vi "read_spectrometer.vi"() -> (0 "spectrometer_data":dbl[][](array[numeric]))   [LabVIEW 2018]
panel:
  out "falling":dbl
  out "FPWM":dbl
  out "rasing":dbl
  out "center wavelength":dbl
  in  "停止":bool
  out "XY Graph":cluster{"Y":dbl[], "Y":dbl[]}[](graph) caption="XY图"
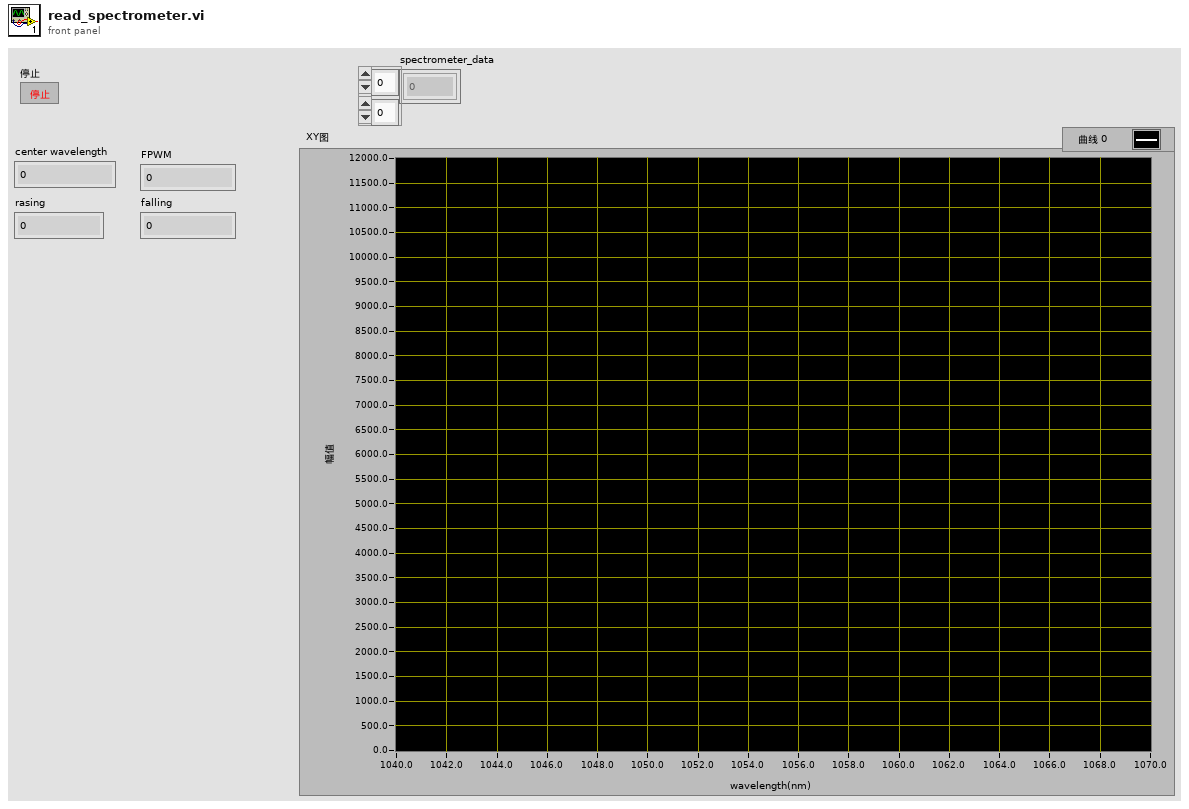
[diagram p1: front panel]
types:
  T1 = enum16{"Read", "Write", "ReadWrite", "BufferedRead", "BufferedReadWrite"}
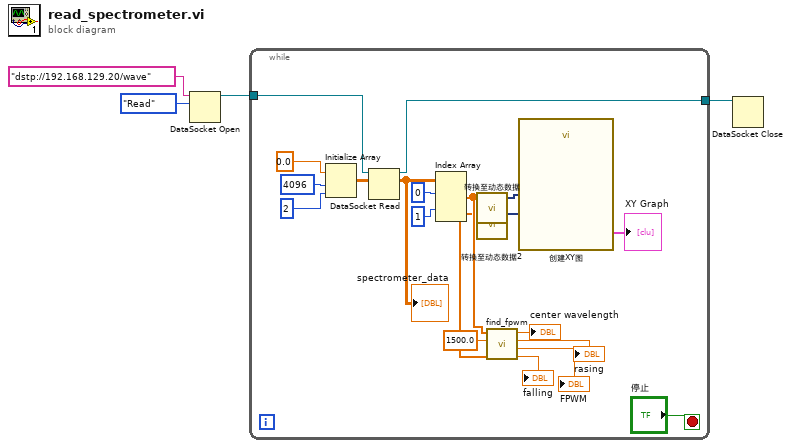
[diagram p0: block diagram]
diagram:
  n1 = DataSocket Open(10:T1."Read" ("模式"), 11:"dstp://192.168.129.20/wave" ("URL")) -> (3:w2:refnum<k13>)  [unwired: 2 in, 1 out]
  n2 = while {
    tunnel: w2 -> [w14]
    tunnel: [w12] -> w1
    stop <- "停止" stop-if-true
    n3 = Initialize Array(0.0 ("元素"), 4096 ("维数大小"), 2 ("维数大小")) -> (w21:dbl[][])
    n4 = DataSocket Read(10:w21, 11:w14) -> (2:w20:dbl[][], 3:w12:refnum<k13>)  [unwired: 3 in, 5 out]
    "spectrometer_data" <- w20
    n5 = Index Array(array=w20, index (row) #1=0 ("索引 (行)"), index (row) #2=1 ("索引 (行)")) -> (element #1=w11:dbl[], element #2=w10:dbl[])  [unwired: 2 in]
    n6 = call "转换至动态数据"("Array"=w11) -> ("Dynamic Data Type"=w16:dynamicdata)  [unwired: 3 in]
    n7 = call "转换至动态数据2"("Array"=w10) -> ("Dynamic Data Type"=w15:dynamicdata)  [unwired: 3 in]
    n8 = call "find_fpwm.vi"("Y"=w10, "baseline"=1500.0, "X"=w11) -> ("falling"=→"falling":dbl, "FPWM"=→"FPWM":dbl, "rasing"=→"rasing":dbl, "center wavelength"=→"center wavelength":dbl)  [unwired: 4 in, 1 out]
    n9 = call "创建XY图"("Y Input"=w15, "X Input"=w16) -> ("XY Graph"=→"XY Graph":cluster{"X":dbl[], "Y":dbl[]}[])  [unwired: 8 in, 1 out]
  }
  n10 = DataSocket Close(11:w1) -> ()  [unwired: 2 in, 2 out]
